vi "Temporary Disable Option.vi"(8 "error in (no error)":errorcluster, 9 "Disable Option (Disable)":i32(ring)=1 items=["Revert Disabling", "Disable"], 10 "Option Name (\"ZNB-K19\")":string="ZNB-K19", 11 "VISA resource name":refnum<visa-resource-name>) -> (0 "error out":errorcluster, 3 "VISA resource name out":refnum<visa-resource-name>)   [LabVIEW 2020, in "Rohde&Schwarz CMXP Base.lvlib"]
doc: "This VI allows a temporary disabling of a named option.\n\nAttribute:\n-\n\nRemote-control command:\nSYSTem:OPTions:DISable"
uses:
  <instrlib>/Rohde&Schwarz CMXP Base/Rohde&Schwarz CMXP Base.lvlib
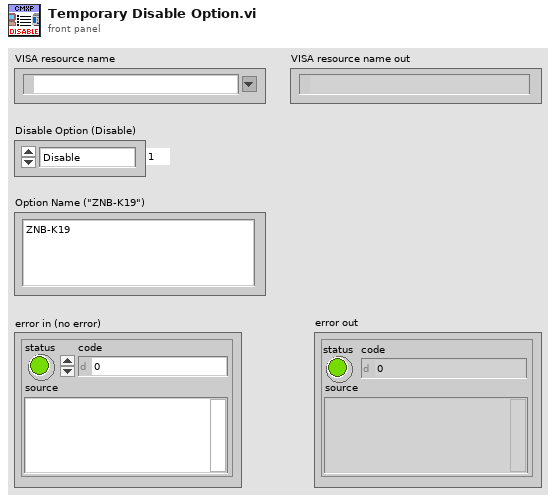
[diagram p1: front panel]
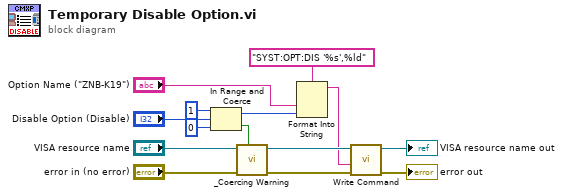
[diagram p0: block diagram]
diagram:
  n1 = In Range and Coerce(upper limit=1, x="Disable Option (Disable)", lower limit=0) -> (coerced(x)=w5:i32, In Range?=w13:bool)
  n2 = call <instrlib>:"_Coercing Warning.vi"("In Range?"=w13, "error in (no error)"="error in (no error)", "VISA resource name"="VISA resource name") -> ("error out"=w11:errorcluster, "VISA resource name out"=w12:refnum<visa-resource-name>)  [unwired: 7 in]
  n3 = Format Into String(format string="SYST:OPT:DIS '%s',%ld", "Option Name (\"ZNB-K19\")", w5) -> (resulting string=w1:string)  [unwired: 2 in, 1 out]
  n4 = call <instrlib>:"Write Command.vi"("error in (no error)"=w11, "Command"=w1, "VISA resource name"=w12) -> ("error out"=→"error out":errorcluster, "VISA resource name out"=→"VISA resource name out":refnum<visa-resource-name>)  [unwired: 7 in]
